vi "testingPID.vi"() -> ()   [LabVIEW 2016]
doc: "Used to tune PID loops"
uses:
  Robot Global Data.vi
panel:
  in  "Slide":dbl(slide)
  in  "FF":dbl
  out "Waveform Chart":dbl(graph)
  in  "Gains":T1={"proportional gain (Kc)"=1.0, "integral time (Ti, min)"=0.0, "derivative time (Td, min)"=0.0} {"derivative time (Td, min)" format="%.5f"; "integral time (Ti, min)" format="%.3f"; "proportional gain (Kc)" format="%.3f"}
  in  "Range":cluster{"output high":dbl, "output low":dbl}={"output high"=0.5, "output low"=-0.5} {"output low" format="%.2f"; "output high" format="%.2f"}
  in  "Chart Slowing":u32(knob)=2 scale=1.0..6.0
  out "Graph":cluster{"B":dbl, dbl}(graph)
  in  "B":dbl=50.0
  in  "A":dbl
  in  "A?":bool
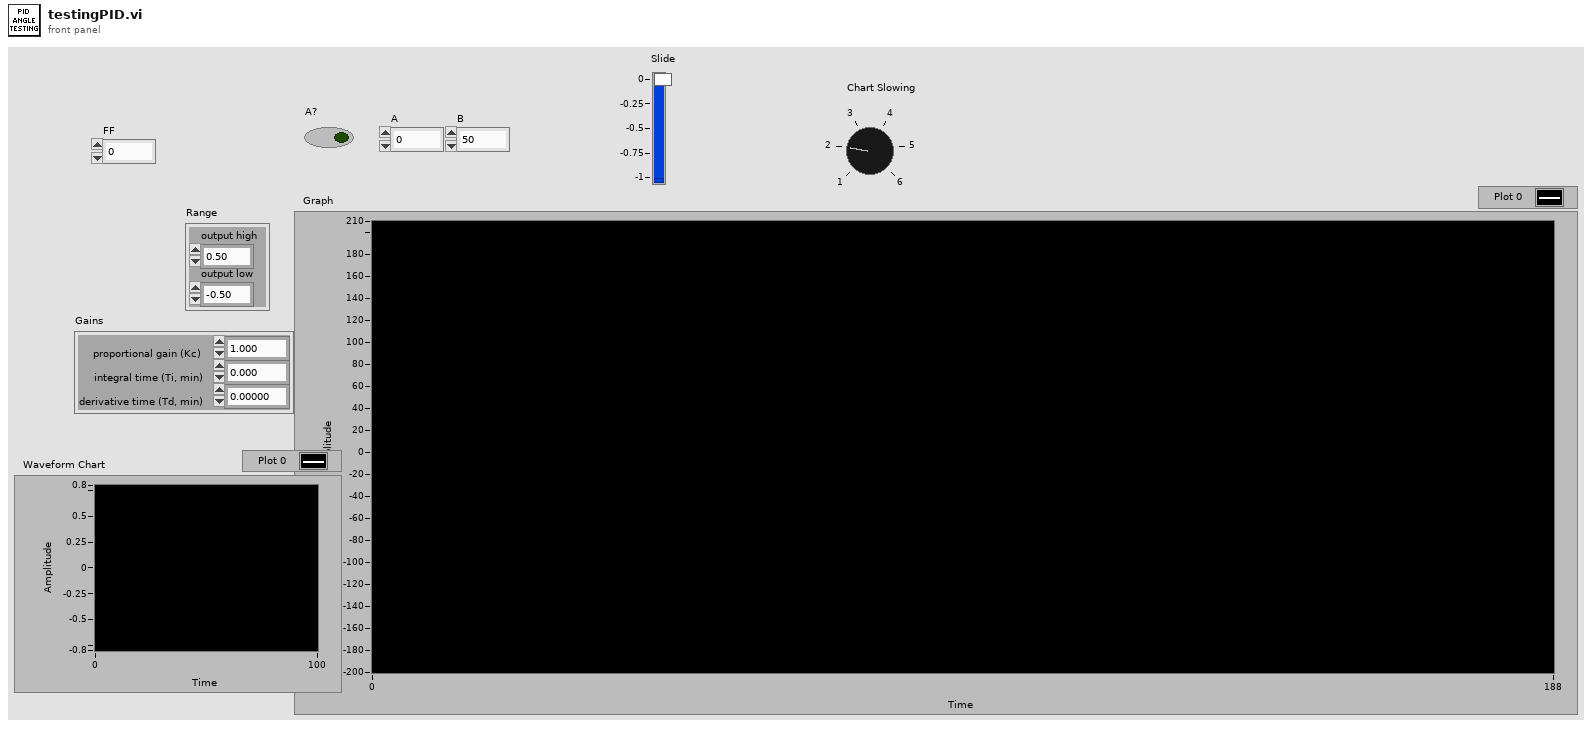
[diagram p1: front panel]
types:
  T1 = cluster{"proportional gain (Kc)":dbl, "integral time (Ti, min)":dbl, "derivative time (Td, min)":dbl}
  T2 = typedef "WPI_EncoderDevRef.ctl" = cluster{"DevStatus":errorcluster, "EncoderIndex":T3, "CounterIndex":T4, "DistancePerCount":dbl, "Decoding Type":T5}
  T3 = typedef "FPGA_EncoderIdx.ctl" = enum8{"Enc 0", "Enc 1", "Enc 2", "Enc 3", "Enc 4", "Enc 5", "Enc 6", "Enc 7", "Invalid"}
  T4 = typedef "FPGA_CounterCtrSystemIndex.ctl" = enum8{"Ctr 0", "Ctr 1", "Ctr 2", "Ctr 3", "Ctr 4", "Ctr 5", "Ctr 6", "Ctr 7", "Invalid"}
  T5 = typedef "WPI_EncoderType.ctl" = enum16{"1x", "2x", "4x"}
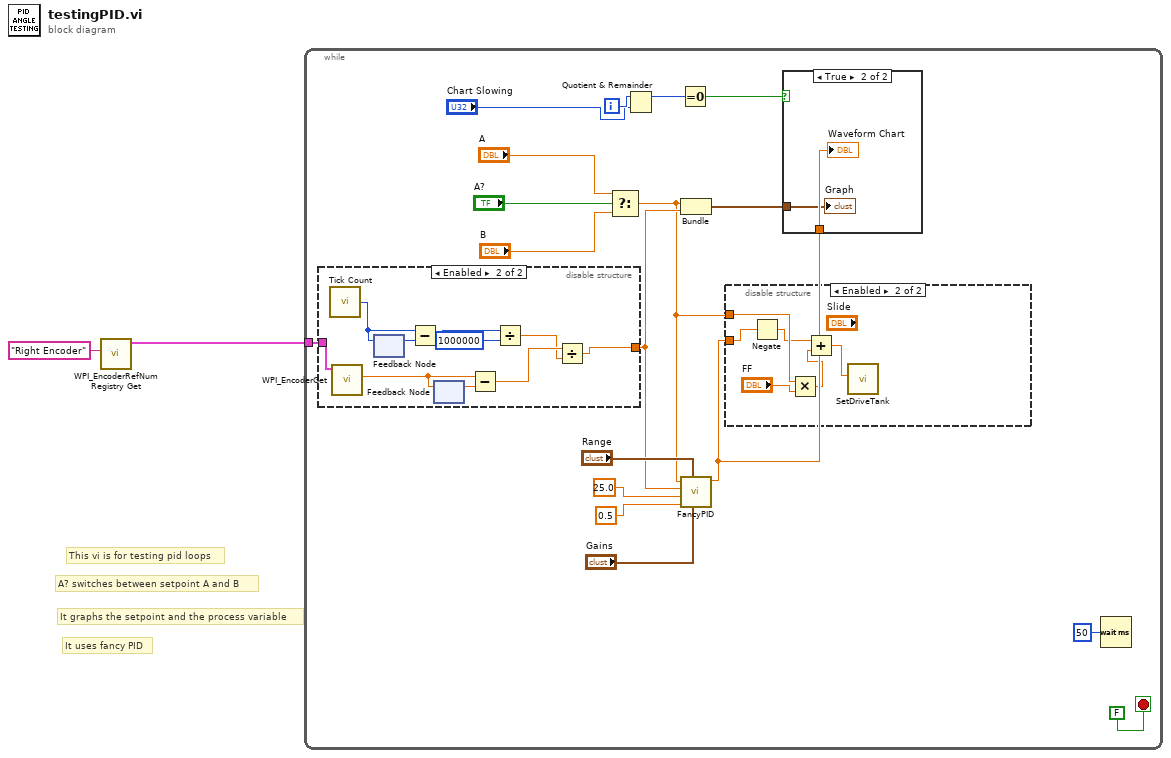
[diagram p0: block diagram]
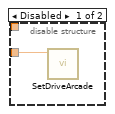
[diagram p2: hidden frame]
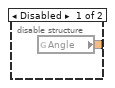
[diagram p3: hidden frame]
diagram:
  # "It uses fancy PID"
  # "It graphs the setpoint and the process variable"
  # "A? switches between setpoint A and B"
  # "This vi is for testing pid loops"
  n1 = call <vilib>:"WPI_EncoderRefNum Registry Get.vi"("refnum name"="Right Encoder") -> ("EncoderDevRef"=w1:T2)  [unwired: 9 in, 1 out]
  n2 = while {
    tunnel: w1 -> [w3]
    i -> [w12]
    stop <- FALSE stop-if-true
    n3 = disable-structure shown="Enabled" {
      disable-tunnel: [w28 w32] -> w8
      disable-tunnel: w3 -> [_ w29]
      frame Disabled {
        n4 = global read "Robot Global Data.vi" "Angle"() -> (w28:dbl)
      }
      frame Enabled {
        n5 = call "Tick Count"() -> ("Tick Count(uSec)"=w31:u32)
        n6 = call <vilib>:"WPI_EncoderGet.vi"("EncoderDevRef"=w29) -> ("Distance"=w30:dbl)  [unwired: 5 in, 5 out]
        n7 = feedback #1() -> (w36:u32)  [unwired: 1 in]
        n8 = feedback-in #1(w31) -> ()
        n9 = Subtract(x=w31, y=w36) -> (x-y=w35:u32)
        n10 = feedback-in #2(w30) -> ()
        n11 = feedback #2() -> (w38:dbl)  [unwired: 1 in]
        n12 = Subtract(x=w30, y=w38) -> (x-y=w37:dbl)
        n13 = Divide(x=w35, y=u32 1000000) -> (x/y=w33:dbl)
        n14 = Divide(x=w37, y=w33) -> (x/y=w32:dbl)
      }
    }
    n15 = Select(t="A", s="A?", f="B") -> (s? t:f=w4:dbl)
    n16 = Quotient & Remainder(x=w12, y="Chart Slowing") -> (x-y*floor(x/y)=w10:u32)  [unwired: 1 out]
    n17 = Equal To 0?(x=w10) -> (x = 0?=w9:bool)
    n18 = Bundle("B"=w4, w8) -> (w7:cluster{"B":dbl, dbl})  [unwired: 1 in]
    n19 = call "FancyPID.vi"("Gains"="Gains", "Range"="Range", "Disable Range"=0.5, "Integral Range"=25.0, "Process variable"=w8, "Setpoint"=w4) -> ("output"=w5:dbl)  [unwired: 5 in]
    n20 = disable-structure shown="Enabled" {
      disable-tunnel: w5 -> [w21 w25]
      disable-tunnel: w4 -> [_ w26]
      frame Disabled {
        n21 = call "SetDriveArcade.vi"("Turn"=w21) -> ()  [unwired: 10 in, 1 out]
      }
      frame Enabled {
        n22 = Negate(x=w25) -> (-x=w24:dbl)
        n23 = Multiply(x=w26, y="FF") -> (x*y=w22:dbl)
        n24 = Add(x=w24, y=w22) -> (x+y=w23:dbl)
        n25 = call "SetDriveTank.vi"("Right"=w23) -> ()  [unwired: 10 in, 1 out]
      }
    }
    n26 = case shown="True" w9 {
      tunnel: w7 -> [_ w39]
      tunnel: w5 -> [_ w40]
      frame False {
      }
      frame True {
        "Graph" <- w39
        "Waveform Chart" <- w40
      }
    }
    n27 = Wait (ms)(milliseconds to wait=u32 50) -> ()  [unwired: 1 out]
  }
